vi "팝업.vi"() -> ()   [LabVIEW 2014]
panel:
  in  "취소 버튼":bool
  in  "확인 버튼":bool
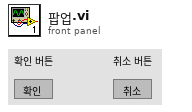
[diagram p1: front panel]
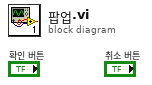
[diagram p0: block diagram]
diagram:
